vi "Create_Partial_SuBUS_Waveform.vi"(0 "OVS":u8=16, 1 "Value":i32=13, 2 "Bit_length":i32=4, 3 "sample rate":dbl=1000.0 format="%#_6p", 5 "error in (no error)":errorcluster) -> (14 "Digital Waveform Graph_Out":digitalwaveform(graph), 19 "error out":errorcluster)   [LabVIEW 2013]
uses:
  <vilib>/Waveform/DWDTOps.llb/DWDT Append Digital Samples.vi
  <vilib>/Waveform/DWDTOps.llb/Digital Pattern Generator (Single Value).vi
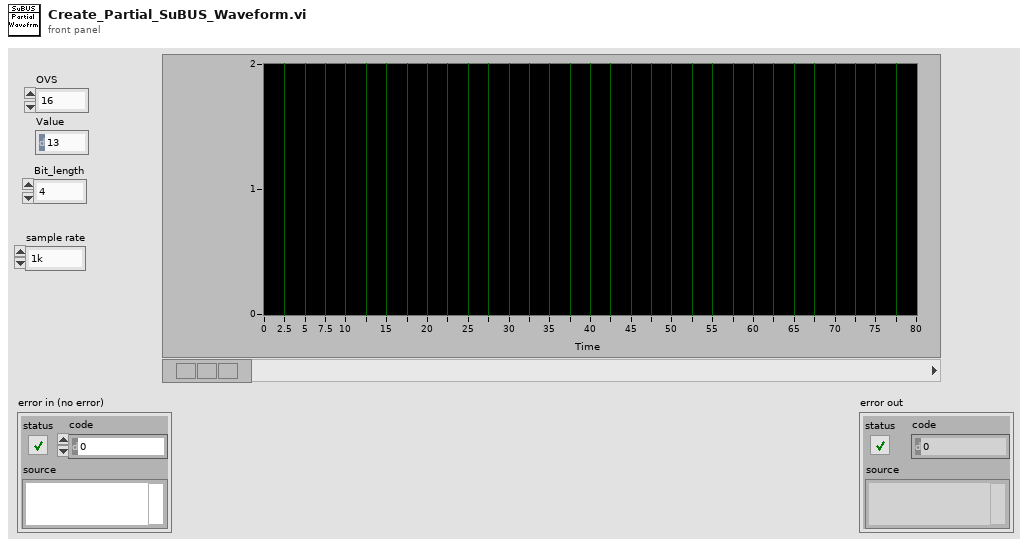
[diagram p1: front panel]
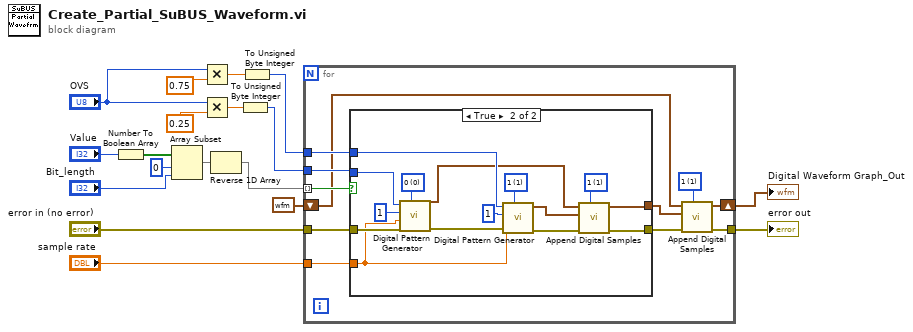
[diagram p0: block diagram]
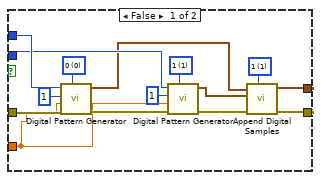
[diagram p2: hidden frame]
diagram:
  n1 = Number To Boolean Array(number="Value") -> (Boolean array=w16:bool[])
  n2 = Array Subset(array=w16, index=0, length="Bit_length") -> (w15:bool[])
  n3 = Multiply(x="OVS", y=0.75) -> (x*y=w12:dbl)
  n4 = Multiply(x="OVS", y=0.25) -> (x*y=w11:dbl)
  n5 = Reverse 1D Array(array=w15) -> (reversed array=w4:bool[])
  n6 = To Unsigned Byte Integer(number=w11) -> (unsigned 8bit integer=w9:u8)
  n7 = To Unsigned Byte Integer(number=w12) -> (unsigned 8bit integer=w10:u8)
  n8 = for {
    tunnel: w4 -> [w27] mode=indexing
    tunnel: w10 -> [w29]
    tunnel: w9 -> [w28]
    shift-right: [w24] -> w3
    shift-left: digitalwaveform {"t0"=timestamp(0 s since 1904-01-01), "dt"=0.0, "Y"={"transitions"=[], "data"=[]}} ("digital waveform out") -> [w20]
    tunnel: "error in (no error)" -> [w22]
    tunnel: [w21] -> w2
    tunnel: "sample rate" -> [w19]
    w23 = u8 1 items=["0", "1", "Z", "L", "H", "X", "T", "V"] ("default value")
    n9 = case shown="True" w27 {
      tunnel: w29 -> [w42 w53]
      tunnel: w28 -> [w37 w54]
      tunnel: [w34 w49] -> w25
      tunnel: [w33 w48] -> w26
      tunnel: w22 -> [w31 w46]
      tunnel: w19 -> [w30 w45]
      frame False {
        w32 = u8 1 items=["0", "1", "Z", "L", "H", "X", "T", "V"] ("default value")
        w40 = u8 1 items=["0", "1", "Z", "L", "H", "X", "T", "V"] ("value")
        w43 = u8 0 items=["0", "1", "Z", "L", "H", "X", "T", "V"] ("value")
        n10 = call-poly <vilib>:"Digital Pattern Generator.vi"("value"=w43, "error in (no error)"=w31, "sample rate"=w30, "number of signals"=u32 1, "number of samples"=w42) -> ("error out"=w39:errorcluster, "digital waveform"=w36:digitalwaveform)  [unwired: 5 in]
        n11 = call-poly <vilib>:"Digital Pattern Generator.vi"("value"=w40, "error in (no error)"=w39, "sample rate"=w30, "number of signals"=u32 1, "number of samples"=w37) -> ("error out"=w38:errorcluster, "digital waveform"=w35:digitalwaveform)  [unwired: 5 in]
        n12 = call-poly <vilib>:"Append Digital Samples.vi"("default value"=w32, "error in (no error)"=w38, "digital waveform B"=w35, "digital waveform A"=w36) -> ("error out"=w33:errorcluster, "digital waveform out"=w34:digitalwaveform)  [unwired: 6 in]
      }
      frame True {
        w47 = u8 1 items=["0", "1", "Z", "L", "H", "X", "T", "V"] ("default value")
        w56 = u8 1 items=["0", "1", "Z", "L", "H", "X", "T", "V"] ("value")
        w59 = u8 0 items=["0", "1", "Z", "L", "H", "X", "T", "V"] ("value")
        n13 = call-poly <vilib>:"Digital Pattern Generator.vi"("value"=w59, "error in (no error)"=w46, "sample rate"=w45, "number of signals"=u32 1, "number of samples"=w54) -> ("error out"=w52:errorcluster, "digital waveform"=w51:digitalwaveform)  [unwired: 5 in]
        n14 = call-poly <vilib>:"Digital Pattern Generator.vi"("value"=w56, "error in (no error)"=w52, "sample rate"=w45, "number of signals"=u32 1, "number of samples"=w53) -> ("error out"=w55:errorcluster, "digital waveform"=w50:digitalwaveform)  [unwired: 5 in]
        n15 = call-poly <vilib>:"Append Digital Samples.vi"("default value"=w47, "error in (no error)"=w55, "digital waveform B"=w50, "digital waveform A"=w51) -> ("error out"=w48:errorcluster, "digital waveform out"=w49:digitalwaveform)  [unwired: 6 in]
      }
    }
    n16 = call-poly <vilib>:"Append Digital Samples.vi"("default value"=w23, "error in (no error)"=w26, "digital waveform B"=w25, "digital waveform A"=w20) -> ("error out"=w21:errorcluster, "digital waveform out"=w24:digitalwaveform)  [unwired: 6 in]
  }
  "Digital Waveform Graph_Out" <- w3
  "error out" <- w2
